vi "Bind To Type - Class - Type Is Same.vi"() -> ()   [LabVIEW 2017, in "Default Serialization Binder Tests.lvlib"]
uses:
  Default Serialization Binder Tests.lvlib
  Class/Class.lvclass
  Default Serialization Binder/Default Serialization Binder.lvclass
  <vilib>/addons/_JKI Toolkits/Caraya/classes/Assert/Assert Equal Value and Type_Variant.vi
  <vilib>/addons/_JKI Toolkits/Caraya/classes/Test/Test.lvclass
  <vilib>/addons/_JKI Toolkits/Caraya/classes/Assert/Assert.lvclass
panel:
  out "error out":errorcluster
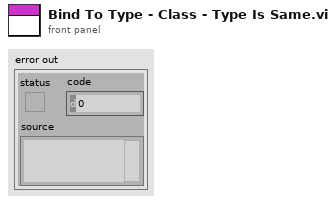
[diagram p1: front panel]
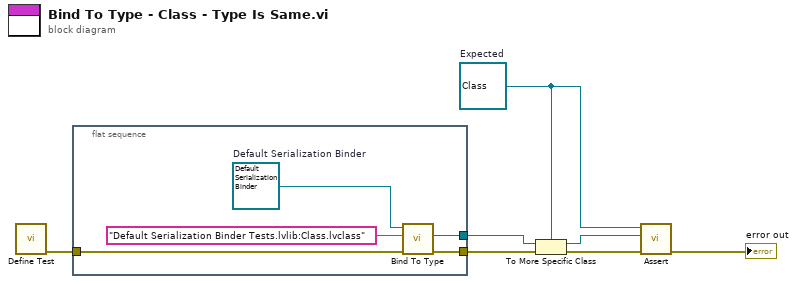
[diagram p0: block diagram]
diagram:
  w2 = refnum<class "Class.lvclass"> refnum  # Expected
  n1 = call <vilib>:"Define Test.vi"() -> ("error out"=w5:errorcluster)  [unwired: 11 in]
  n2 = flat-sequence {
    tunnel: [w10] -> w3
    tunnel: [w8] -> w6
    tunnel: w5 -> [w9]
    frame #0 {
      w12 = refnum<class "Default Serialization Binder.lvclass"> refnum  # Default Serialization Binder
      n3 = call-dynamic "Bind To Type.vi"("error in (no error)"=w9, "Type Name"="Default Serialization Binder Tests.lvlib:Class.lvclass", "Default Serialization Binder in"=w12) -> ("error out"=w8:errorcluster, "Type"=w10:refnum<class>)  [unwired: 6 in, 1 out]
    }
  }
  n4 = To More Specific Class(target class=w2, reference=w3, error in=w6) -> (specific class reference=w1:refnum<class "Class.lvclass">, error out=w4:errorcluster)
  n5 = call-poly <vilib>:"Assert.vi"("error in (no error)"=w4, "Y"=w1, "X"=w2) -> ("error out"=→"error out":errorcluster)  [unwired: 8 in]
